vi "Data Execute (Tree).vi"(8 "error in (no error)":errorcluster, 9 "Tree in":refnum<data-value>, 10 "Expression":string, 11 "Data DVR in":refnum<data-value>) -> (0 "error out":errorcluster, 1 "Tree out":refnum<data-value>, 2 "Data out":refnum<data-value>, 3 "Data DVR out":refnum<data-value>)   [LabVIEW 2012, in "MDSplus.lvlib"]
doc: "Compile and evaluate expression."
uses:
  <vilib>/MDSplus/Library/MDSplus.lvlib
  <vilib>/MDSplus/Classes/Tree_Class/Tree.lvclass
  <vilib>/MDSplus/Classes/Data_Class/Data.lvclass
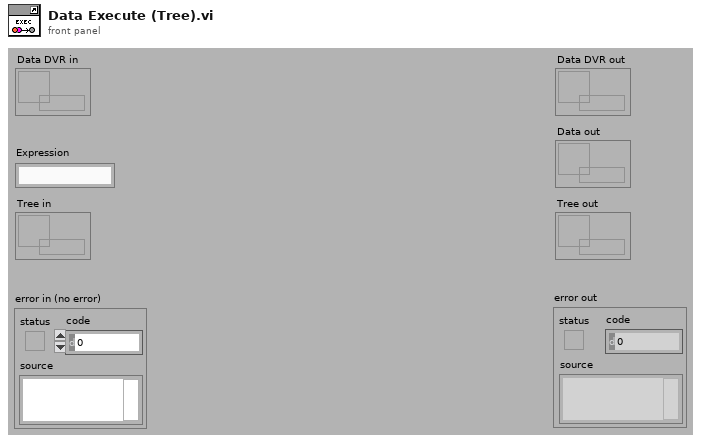
[diagram p1: front panel]
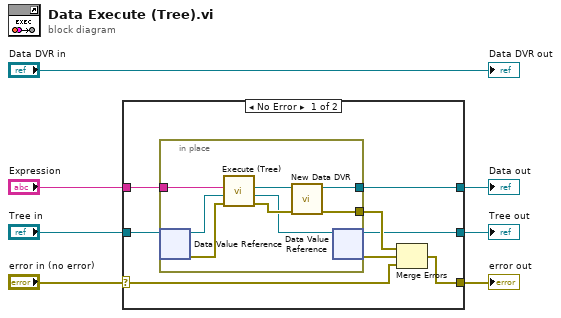
[diagram p0: block diagram]
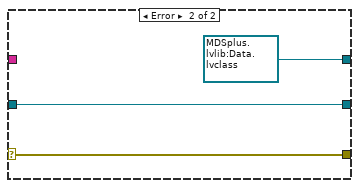
[diagram p2: hidden frame]
diagram:
  n1 = case shown="No Error" "error in (no error)" {
    selector: "error in (no error)" -> [w15 w26]
    tunnel: [w14 w26] -> w4
    tunnel: [w11 refnum<data-value> refnum ("TreeNode DVR out")] -> w2
    tunnel: "Expression" -> [w13 _]
    tunnel: "Tree in" -> [w12 w24]
    tunnel: [w8 w24] -> w3
    frame No Error {
      n2 = in-place {
        in-place-border: [w22] -> w10
        in-place-border: w13 -> [w16]
        in-place-border: [w23] -> w11
        n3 = in-place-dvr #1(w12) -> (w19:refnum<class "Tree.lvclass">, w21:errorcluster)
        n4 = call <vilib>:"Execute (Tree).vi"("error in (no error)"=w21, "Tree in"=w19, "Expression"=w16) -> ("error out"=w20:errorcluster, "Tree out"=w18:refnum<class "Tree.lvclass">, "Returned data out"=w17:refnum<class "Data.lvclass">)  [unwired: 5 in, 1 out]
        n5 = call <vilib>:"New Data DVR.vi"("error in (no error)"=w20, "Data in"=w17) -> ("error out"=w22:errorcluster, "Data DVR out"=w23:refnum<data-value>)  [unwired: 8 in]
        n6 = in-place-dvr #1(w18) -> (w8:refnum<data-value>, w9:errorcluster)
      }
      n7 = Merge Errors(w10, w9, w15) -> (w14:errorcluster)
    }
    frame Error {
    }
  }
  "error out" <- w4
  "Tree out" <- w3
  "Data out" <- w2
  "Data DVR out" <- "Data DVR in"
